vi "2 PureWaypointHeadingGoodness.vi"(3 "Waypoint Location":T1 {"North" format="%#_10f"; "East" format="%#_8f"}, 4 "Heading to Test":dbl) -> (1 "Goodness":dbl)   [LabVIEW 2011]
doc: "Takes the absolute wind vector, the heading of your next waypoint, and a test heading and outputs a goodness value for the test heading. The criteria is the speed to get to the waypoint.\n\nThe goodness is evaluated by taking the softmax of an angle with all possible complimenting angles (i.e. if the test heading is 10 degrees it is matched with -1 through -89; note that angles are adjusted to be degrees from directly at the waypoint). The specific calculation for finding the net velocity of a pair of angles requires the velocities from the polar plot."
uses:
  2 Typedefs/UTM Location.ctl
  2 Globals/2 Global.vi
panel:
  out "Heading to Waypt":dbl
  # "Inputs"
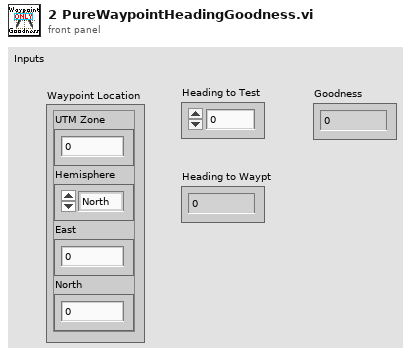
[diagram p1: front panel]
types:
  T1 = typedef "UTM Location.ctl" = cluster{"UTM Zone":dbl, "Hemisphere":enum16{"North", "South"}, "East":dbl, "North":dbl}
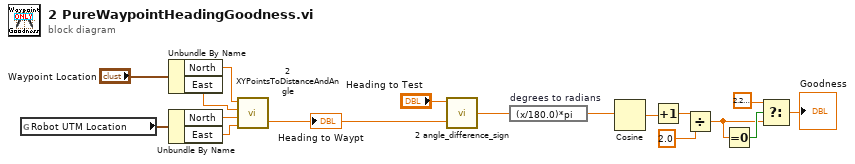
[diagram p0: block diagram]
diagram:
  n1 = global read "2 Global.vi" "Robot UTM Location"() -> (w10:T1)
  n2 = Unbundle By Name("Waypoint Location") -> ("North"=w12:dbl, "East"=w11:dbl)
  n3 = Unbundle By Name(w10) -> ("North"=w13:dbl, "East"=w14:dbl)
  n4 = call "2 XYPointsToDistanceAndAngle.vi"("East 2"=w14, "North 2"=w13, "East 1"=w11, "North 1"=w12) -> ("Angle Diff"=w7:dbl)  [unwired: 1 out]
  "Heading to Waypt" <- w7
  n5 = call "2 angle_difference_sign.vi"("Angle 2"=w7, "Angle 1"="Heading to Test") -> ("Difference"=w5:dbl)
  n6 = expression code="(x/180.0)*pi" "degrees to radians"(w5) -> (w6:dbl)
  n7 = Cosine(x=w6) -> (cos(x)=w4:dbl)
  n8 = Increment(x=w4) -> (x+1=w3:dbl)
  n9 = Divide(x=w3, y=2.0) -> (x/y=w1:dbl)
  n10 = Equal To 0?(x=w1) -> (x = 0?=w8:bool)
  n11 = Select(t=2.220446049250313e-16, s=w8, f=w1) -> (s? t:f=→"Goodness":dbl)
